vi "Get DAQ Settings.vi"(8 "error in (no error)":errorcluster, 10 "Physical Chan Array":i32[](array[numeric]), 11 "Device Ref in":T1 format="%.0x") -> (0 "error out":errorcluster, 2 "DAQ Config Data":T2, 3 "Device Ref Out":T1 format="%.0x")   [LabVIEW 2020, in "Waveform Analog Output Engine.lvlib"]
doc: "Reads all of the DAQ configuration properties from the custom device"
uses:
  Waveform Analog Output Engine.lvlib
  <vilib>/NI VeriStand/Custom Device API/Custom Device Item Ref.ctl
  DAQ Config Data.ctl
  Shared/Constants.vi
  <vilib>/NI VeriStand/Custom Device API/Get Item Property (String).vi
  <vilib>/NI VeriStand/Custom Device API/Get Item Property (Double).vi
  <vilib>/NI VeriStand/Custom Device API/Get Item Property (U32).vi
  <vilib>/NI VeriStand/Custom Device API/Custom Device API.lvlib
  Shared/Waveform Analog Output Shared.lvlib
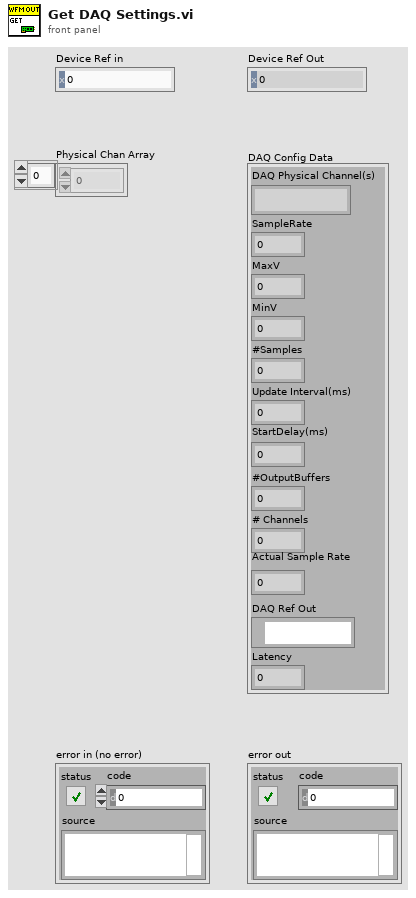
[diagram p1: front panel]
types:
  T1 = typedef "Custom Device API.lvlib/Custom Device Item Ref.ctl" = u64
  T2 = typedef "Waveform Analog Output Engine.lvlib/DAQ Config Data.ctl" = cluster{"DAQ Physical Channel(s)":string, "SampleRate":dbl, "MaxV":dbl, "MinV":dbl, "#Samples":dbl, "Update Interval(ms)":u32, "StartDelay(ms)":dbl, "#OutputBuffers":dbl, "# Channels":i32, "Actual Sample Rate":dbl, "DAQ Ref Out":refnum<k21>, "Latency":dbl}
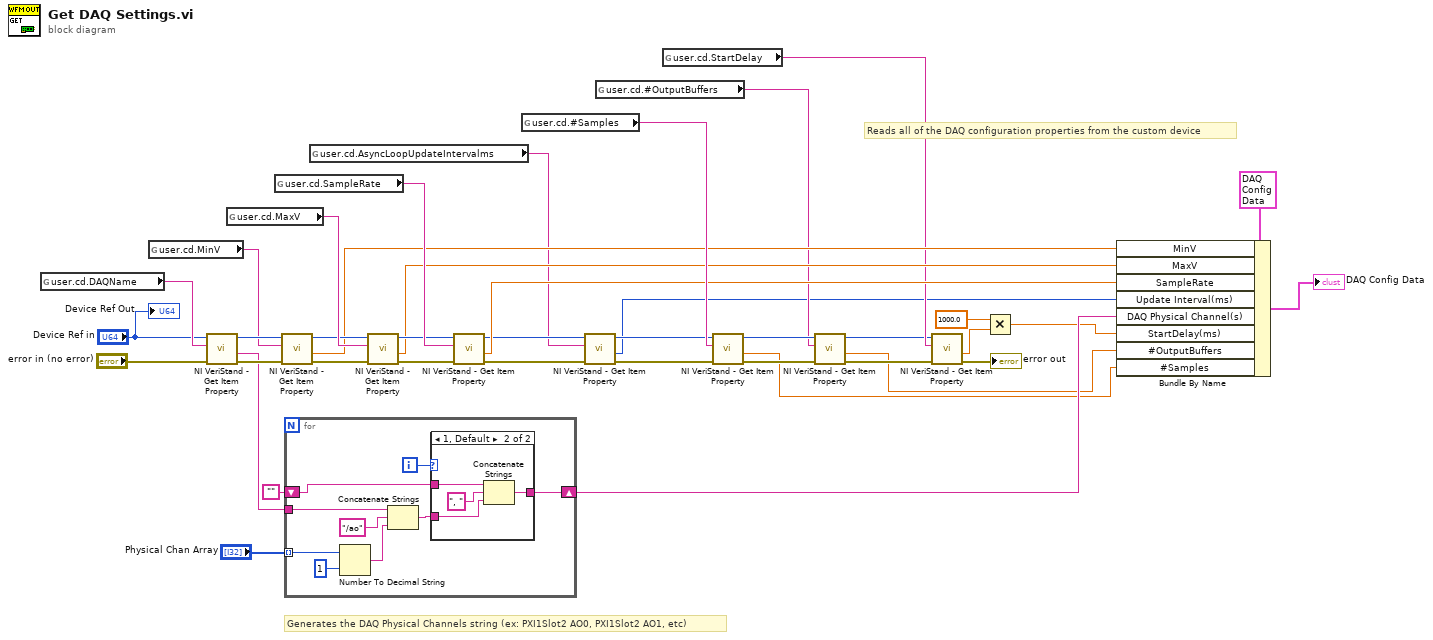
[diagram p0: block diagram]
diagram:
  # "Generates the DAQ Physical Channels string (ex: PXI1Slot2 AO0, PXI1Slot2 AO1, etc)"
  # "Reads all of the DAQ configuration properties from the custom device"
  n1 = global read "Constants.vi" "user.cd.DAQName"() -> (w38:string)
  n2 = global read "Constants.vi" "user.cd.MinV"() -> (w29:string)
  n3 = call-poly <vilib>:"NI VeriStand - Get Item Property.vi"("error in (no error)"="error in (no error)", "Property Name"=w38, "Item Ref in"="Device Ref in") -> ("error out"=w35:errorcluster, "Value"=w26:string, "Item Ref out"=w34:T1)  [unwired: 5 in, 1 out]
  n4 = global read "Constants.vi" "user.cd.MaxV"() -> (w30:string)
  n5 = global read "Constants.vi" "user.cd.SampleRate"() -> (w33:string)
  n6 = call-poly <vilib>:"NI VeriStand - Get Item Property.vi"("error in (no error)"=w35, "Property Name"=w29, "Item Ref in"=w34) -> ("error out"=w28:errorcluster, "Value"=w23:dbl, "Item Ref out"=w27:T1)  [unwired: 5 in, 1 out]
  n7 = for {
    tunnel: w26 -> [w47]
    shift-right: [w42] -> w20
    shift-left: "" -> [w41]
    tunnel: "Physical Chan Array" -> [w46] mode=indexing
    i -> [w49]
    n8 = Number To Decimal String(number=w46, width (-)=i16 1) -> (decimal integer string=w44:string)
    n9 = Concatenate Strings(w47, "/ao" ("string"), w44) -> (w43:string)
    n10 = case shown="1, Default" w49 {
      tunnel: w43 -> [w50 w53]
      tunnel: [w50 w52] -> w42
      tunnel: w41 -> [_ w51]
      frame 0 {
      }
      frame 1, Default {
        n11 = Concatenate Strings(w51, ", " ("string"), w53) -> (w52:string)
      }
    }
  }
  n12 = global read "Constants.vi" "user.cd.AsyncLoopUpdateIntervalms"() -> (w2:string)
  n13 = call-poly <vilib>:"NI VeriStand - Get Item Property.vi"("error in (no error)"=w28, "Property Name"=w30, "Item Ref in"=w27) -> ("error out"=w32:errorcluster, "Value"=w22:dbl, "Item Ref out"=w31:T1)  [unwired: 5 in, 1 out]
  n14 = call-poly <vilib>:"NI VeriStand - Get Item Property.vi"("error in (no error)"=w32, "Property Name"=w33, "Item Ref in"=w31) -> ("error out"=w5:errorcluster, "Value"=w21:dbl, "Item Ref out"=w6:T1)  [unwired: 5 in, 1 out]
  n15 = global read "Constants.vi" "user.cd.#Samples"() -> (w25:string)
  n16 = call-poly <vilib>:"NI VeriStand - Get Item Property.vi"("error in (no error)"=w5, "Property Name"=w2, "Item Ref in"=w6) -> ("error out"=w4:errorcluster, "Value"=w1:u32, "Item Ref out"=w3:T1)  [unwired: 5 in, 1 out]
  n17 = global read "Constants.vi" "user.cd.#OutputBuffers"() -> (w12:string)
  n18 = global read "Constants.vi" "user.cd.StartDelay"() -> (w17:string)
  n19 = call-poly <vilib>:"NI VeriStand - Get Item Property.vi"("error in (no error)"=w4, "Property Name"=w25, "Item Ref in"=w3) -> ("error out"=w13:errorcluster, "Value"=w7:dbl, "Item Ref out"=w14:T1)  [unwired: 5 in, 1 out]
  n20 = call-poly <vilib>:"NI VeriStand - Get Item Property.vi"("error in (no error)"=w13, "Property Name"=w12, "Item Ref in"=w14) -> ("error out"=w10:errorcluster, "Value"=w8:dbl, "Item Ref out"=w11:T1)  [unwired: 5 in, 1 out]
  n21 = call-poly <vilib>:"NI VeriStand - Get Item Property.vi"("error in (no error)"=w10, "Property Name"=w17, "Item Ref in"=w11) -> ("error out"=→"error out":errorcluster, "Value"=w16:dbl)  [unwired: 5 in, 2 out]
  n22 = Multiply(x=1000.0, y=w16) -> (x*y=w9:dbl)
  n23 = Bundle By Name(cluster=T2 {"DAQ Physical Channel(s)"="", "SampleRate"=0.0, "MaxV"=0.0, "MinV"=0.0, "#Samples"=0.0, "Update Interval(ms)"=0, "StartDelay(ms)"=0.0, "#OutputBuffers"=0.0, "# Channels"=0, "Actual Sample Rate"=0.0, "DAQ Ref Out"="", "Latency"=0.0} ("DAQ Config Data"), "MinV"=w23, "MaxV"=w22, "SampleRate"=w21, "Update Interval(ms)"=w1, "DAQ Physical Channel(s)"=w20, "StartDelay(ms)"=w9, "#OutputBuffers"=w8, "#Samples"=w7) -> (→"DAQ Config Data":T2)
  "Device Ref Out" <- "Device Ref in"
